vi "Write Page Size.vi"(8 "error in (no error)":errorcluster, 10 "PageSize":dbl, 11 "Scrollbar.lvclass in":refnum<class "Scrollbar.lvclass">) -> (0 "error out":errorcluster, 3 "Scrollbar.lvclass out":refnum<class "Scrollbar.lvclass">)   [LabVIEW 2015, in "Scrollbar.lvclass"]
uses:
  Scrollbar.lvclass
  Scrollbar.lvclass/Scrollbar.ctl
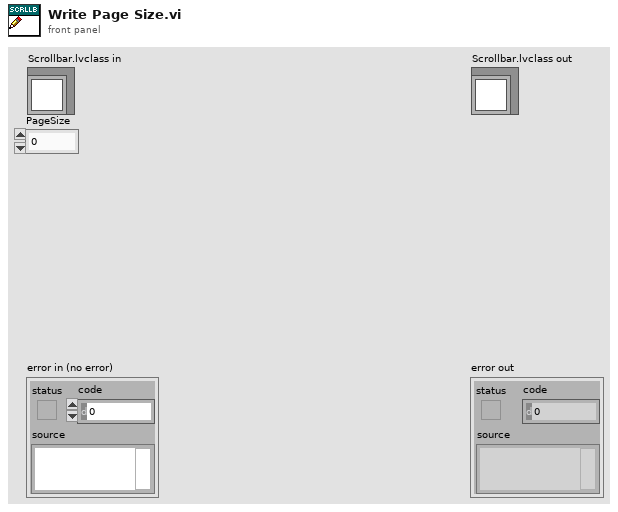
[diagram p1: front panel]
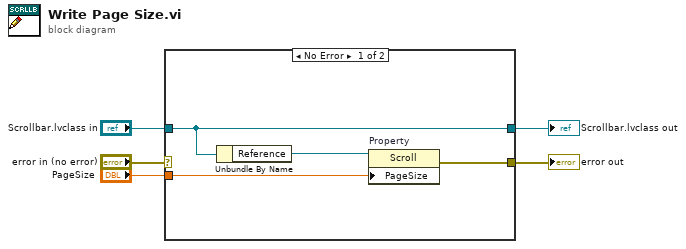
[diagram p0: block diagram]
diagram:
  n1 = case shown="No Error" "error in (no error)" {
    selector: "error in (no error)" -> [_ w11]
    tunnel: [w9 w11] -> w4
    tunnel: [w7 w10] -> w2
    tunnel: "Scrollbar.lvclass in" -> [w7 w10]
    tunnel: "PageSize" -> [w8 _]
    frame No Error {
      n2 = Unbundle By Name(w7) -> ("Reference"=w6:refnum<vi>)
      n3 = property on="Property" class="Scroll"(reference=w6, "PageSize"=w8) -> (error out=w9:errorcluster)  [unwired: 1 in, 1 out]
    }
    frame Error {
    }
  }
  "error out" <- w4
  "Scrollbar.lvclass out" <- w2
